vi "Cylinder.vi"(4 "Position":cluster{"X":sgl, "Y":sgl, "Z":sgl}, 5 "Alpha":dbl=1.0, 6 "Detail":sgl=1.0, 7 "Color Box":u32(colorbox), 8 "error in (no error)":errorcluster, 9 "Size":cluster{"Height":sgl, "Radius":sgl}={"Height"=1.0, "Radius"=1.0}, 10 "Name":string) -> (0 "error out":errorcluster, 3 "3D Object out":refnum<class "3D Object.lvclass">)   [LabVIEW 2015, in "3D Object.lvclass"]
uses:
  3D Object.lvclass
  <vilib>/picture/3D Picture Control/NI_3D Picture Control.lvlib
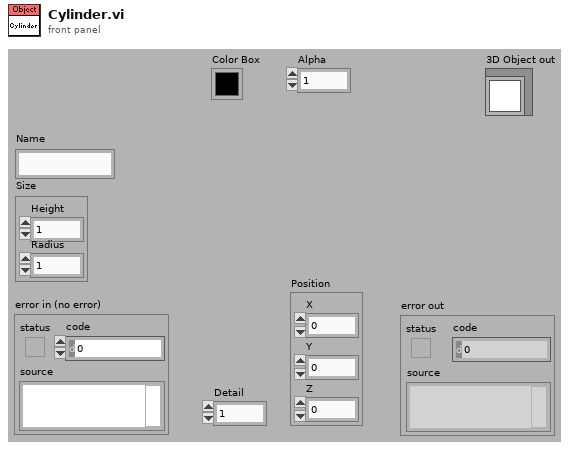
[diagram p1: front panel]
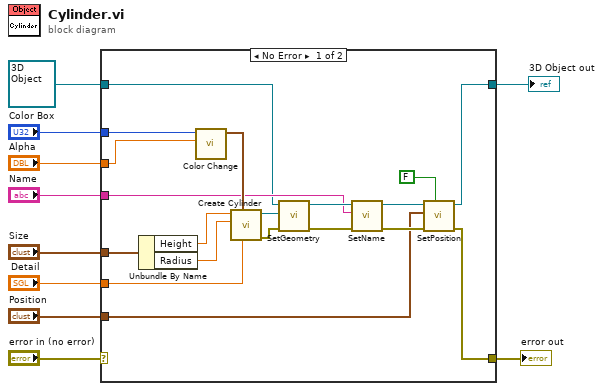
[diagram p0: block diagram]
diagram:
  n1 = case shown="No Error" "error in (no error)" {
    selector: "error in (no error)" -> [_ w31]
    tunnel: "Detail" -> [w29 _]
    tunnel: "Color Box" -> [w28 _]
    tunnel: [w22 w31] -> w7
    tunnel: "Alpha" -> [w24 _]
    tunnel: refnum<class "3D Object.lvclass"> refnum ("3D Object in") -> [w13 w30]
    tunnel: [w23 w30] -> w4
    tunnel: "Position" -> [w12 _]
    tunnel: "Size" -> [w21 _]
    tunnel: "Name" -> [w14 _]
    frame No Error {
      n2 = Unbundle By Name(w21) -> ("Height"=w20:sgl, "Radius"=w19:sgl)
      n3 = call <vilib>:"Color Change.vi"("Alpha"=w24, "Color"=w28) -> ("RGBA"=w27:cluster{"R":sgl, "G":sgl, "B":sgl, "A":sgl})  [unwired: 9 out]
      n4 = call <vilib>:"Create Cylinder.vi"("Detail"=w29, "Color"=w27, "Radius"=w19, "Height"=w20) -> ("error out"=w25:errorcluster, "New Cylinder Refnum"=w26:refnum<vi>)  [unwired: 1 in, 5 out]
      n5 = call "SetGeometry.vi"("error in (no error)"=w25, "Geometry"=w26, "Object in"=w13) -> ("error out"=w17:errorcluster, "Object out"=w18:refnum<class "3D Object.lvclass">)  [unwired: 7 out]
      n6 = call "SetName.vi"("error in (no error)"=w17, "Name"=w14, "3D Object in"=w18) -> ("error out"=w15:errorcluster, "3D Object out"=w16:refnum<class "3D Object.lvclass">)  [unwired: 7 out]
      n7 = call "SetPosition.vi"("Relative?"=FALSE, "error in (no error)"=w15, "Position"=w12, "3D Object in"=w16) -> ("error out"=w22:errorcluster, "3D Object out"=w23:refnum<class "3D Object.lvclass">)  [unwired: 6 in]
    }
    frame Error {
    }
  }
  "error out" <- w7
  "3D Object out" <- w4
